vi "Calculate Position Orientation 2.vi"(8 "error in":errorcluster, 10 "Measured Global Positions":T2(array[cluster]), 11 "Known Local Positions":T2(array[cluster])) -> (0 "error out":errorcluster, 1 "Residual":dbl, 3 "PositionOrientation":T1)   [LabVIEW 2017]
uses:
  Vec3d Class/Vec3d.lvclass
  Type Definitions/Position_Orientation.ctl
  Orient3d Class/Orient3d.lvclass
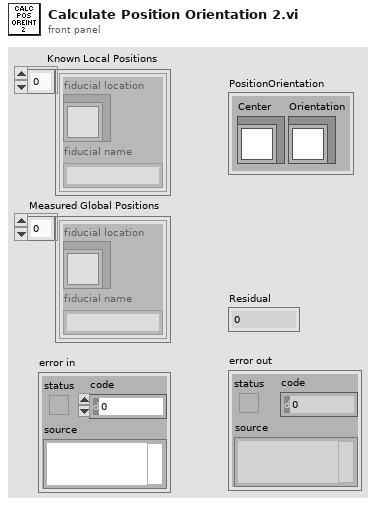
[diagram p1: front panel]
types:
  T1 = typedef "Position_Orientation.ctl" = cluster{"Center":refnum<class "Vec3d.lvclass">, "Orientation":refnum<class "Orient3d.lvclass">}
  T2 = cluster{"fiducial location":refnum<class "Vec3d.lvclass">, "fiducial name":string}[]
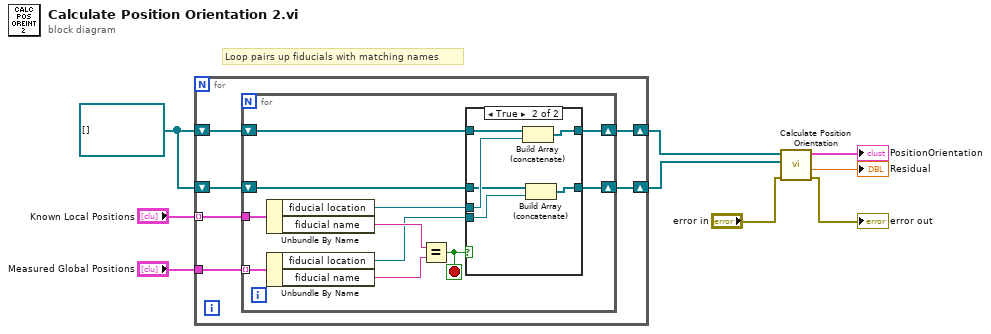
[diagram p0: block diagram]
diagram:
  w9 = refnum<class "Vec3d.lvclass">[] [] ("Known Local Positions")
  # "Loop pairs up fiducials with matching names"
  n1 = for {
    shift-right: [w13] -> w6
    shift-left: w9 -> [w15]
    shift-right: [w12] -> w5
    shift-left: w9 -> [w14]
    tunnel: "Known Local Positions" -> [w11] mode=indexing
    tunnel: "Measured Global Positions" -> [w10]
    n2 = for {
      shift-right: [w18] -> w13
      shift-left: w15 -> [w20]
      shift-right: [w17] -> w12
      shift-left: w14 -> [w19]
      tunnel: w11 -> [w26]
      tunnel: w10 -> [w25] mode=indexing
      stop <- w16 stop-if-true
      n3 = Unbundle By Name(w26) -> ("fiducial location"=w21:refnum<class "Vec3d.lvclass">, "fiducial name"=w23:string)
      n4 = Unbundle By Name(w25) -> ("fiducial location"=w22:refnum<class "Vec3d.lvclass">, "fiducial name"=w24:string)
      n5 = Equal?(x=w23, y=w24) -> (x = y?=w16:bool)
      n6 = case shown="True" w16 {
        tunnel: w22 -> [_ w30]
        tunnel: w21 -> [_ w33]
        tunnel: w20 -> [w28 w34]
        tunnel: w19 -> [w27 w31]
        tunnel: [w28 w32] -> w18
        tunnel: [w27 w29] -> w17
        frame False {
        }
        frame True {
          n7 = Build Array (concatenate)(w34, w33) -> (w32:refnum<class "Vec3d.lvclass">[])
          n8 = Build Array (concatenate)(w31, w30) -> (w29:refnum<class "Vec3d.lvclass">[])
        }
      }
    }
  }
  n9 = call "Calculate Position Orientation.vi"("error in"="error in", "Measured Global Positions"=w5, "Known Local Positions"=w6) -> ("error out"=→"error out":errorcluster, "Residual"=→"Residual":dbl, "PositionOrientation"=→"PositionOrientation":T1)  [unwired: 6 in]
